vi "DAC_set_slot.vi"(8 "DAC Offset":T1 min=-1 max=0.5, 9 "FastChanNumber":u8, 10 "slot number":u16, 11 "FPGA VI Reference In":T2) -> (3 "FPGA VI Reference Out":T2)   [LabVIEW 2013]
uses:
  fpga-bitfile-ref.ctl
  sequence slot/DAC_fastseq-offset.ctl
  slot-use-values.ctl
  slot-use-type.ctl
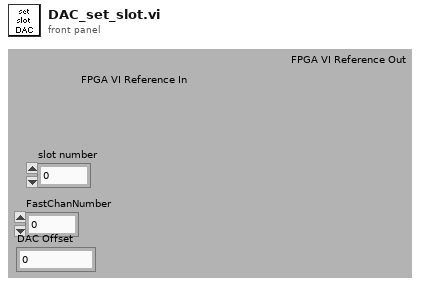
[diagram p1: front panel]
types:
  T1 = typedef "DAC_fastseq-offset.ctl" = sgl
  T2 = typedef "fpga-bitfile-ref.ctl" = refnum<k20>
  T3 = typedef "slot-use-type.ctl" = fxp<+,4,4>
  T4 = typedef "slot-use-values.ctl" = enum16{"DAC", "timing", "triggers", "jump"}
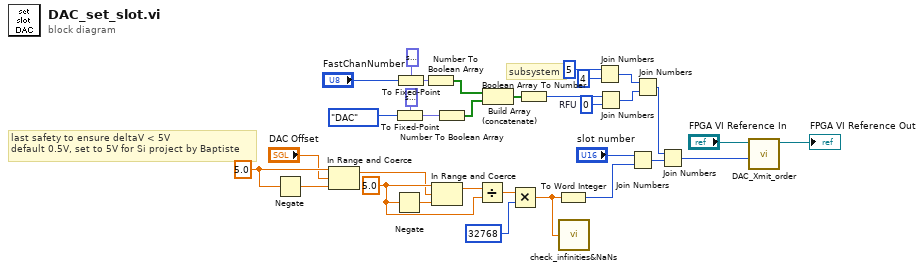
[diagram p0: block diagram]
diagram:
  w15 = T1 5.0 ("upper limit")
  w20 = sgl 5.0 ("y")
  w29 = u8 0  # RFU
  # "last safety to ensure deltaV < 5V\ndefault 0.5V, set to 5V for Si project by Baptiste"
  # "subsystem"
  n1 = Negate(x=w15) -> (-x=w14:T1)
  n2 = In Range and Coerce(upper limit=w15, x="DAC Offset", lower limit=w14) -> (coerced(x)=w13:T1)  [unwired: 1 out]
  n3 = Negate(x=w20) -> (-x=w19:sgl)
  n4 = To Fixed-Point(fixed-point type=T3 0.0, number=slot-use-values."DAC") -> (fixed-point=w11:T3)
  n5 = To Fixed-Point(fixed-point type=T3 0.0, number="FastChanNumber") -> (fixed-point=w21:T3)
  n6 = Number To Boolean Array(number=w21) -> (Boolean array=w1:bool[])
  n7 = In Range and Coerce(upper limit=w20, x=w13, lower limit=w19) -> (coerced(x)=w18:T1)  [unwired: 1 out]
  n8 = Number To Boolean Array(number=w11) -> (Boolean array=w2:bool[])
  n9 = Divide(x=w18, y=w20) -> (x/y=w16:T1)
  n10 = Build Array (concatenate)(w1, w2) -> (w22:bool[])
  n11 = Multiply(x=w16, y=u16 32768) -> (x*y=w12:T1)
  n12 = Boolean Array To Number(Boolean array=w22) -> (number=w4:u8)
  n13 = To Word Integer(number=w12) -> (16bit integer=w3:i16)
  n14 = call "check_infinities&NaNs.vi"("Value"=w12) -> ()
  n15 = Join Numbers(hi=u8 5, lo=u8 4) -> ((hi.lo)=w27:u16)
  n16 = Join Numbers(hi=w4, lo=w29) -> ((hi.lo)=w28:u16)
  n17 = Join Numbers(hi="slot number", lo=w3) -> ((hi.lo)=w25:u32)
  n18 = Join Numbers(hi=w27, lo=w28) -> ((hi.lo)=w24:u32)
  n19 = Join Numbers(hi=w24, lo=w25) -> ((hi.lo)=w32:u64)
  n20 = call "DAC_Xmit_order.vi"("Order in"=w32, "FPGA VI Reference In"="FPGA VI Reference In") -> ("FPGA VI Reference Out"=→"FPGA VI Reference Out":T2)  [unwired: 9 out]
